vi "oa_Build Spectral Info (N Channels).vi"(0 "spectra in":dbl[][][](array[numeric]) format="%.2f", 1 "processing control in":T1(ring), 5 "channel info":T8[](array[typedef]) {"channel info"."pregain" format="%.2f"; "channel info"."weighting filter" items=["Linear", "A-weighting", "B-weighting", "C-weighting", "ITU-R 468-4", "Dolby", "CCITT", "C-message", "Wb", "Wc", "Wd", "We", "Wf", "Wh", "Wj", "Wk", "Wm", "AES17 20 kHz lowpass", "AES17 40 kHz lowpass", "AES17 20 kHz highpass", "AES17 40 kHz highpass"]; "channel info"."dB reference" format="%^.1e"; "channel info"."engineering units" items=["custom..."=0, "V"=1, "A"=21, "C"=30, "pC"=31, "s"=32, "-"=29, "Pa"=2, "N"=20, "g"=3, "m/s^2"=4, "m/s"=5, "m"=6, "mm/s"=12, "mm"=13, "micron/s"=14, "micron"=15, "in/s^2"=7, "in/s"=8, "in"=9, "mil/s"=10, "mil"=11, "rad/s^2"=16, "rad/s"=17, "rad"=18, "deg/s^2"=26, "deg/s"=27, "deg"=28, "RPM"=22, "cycle/s^2"=23, "Hz"=24, "cycle"=25, "strain"=19]; "channel info"."sensor sensitivity" format="%#_5f"}, 7 "spectrum settings":cluster{"window type":u16, "block size":i32}={"window type"=1, "block size"=400} {"block size" min=2; "window type" items=["None"=0, "Hanning"=1, "Hamming"=2, "Blackman-Harris"=3, "Exact Blackman"=4, "Blackman"=5, "Flat Top"=6, "4 Term B-Harris"=7, "7 Term B-Harris"=8, "Low Sidelobe"=9, "Gaussian"=62]}, 11 "error in":errorcluster, 12 "spectrum type":T4=enum."Power [Magnitude^2]") -> (2 "spectrum info":T2[](array[typedef]) {"x-axis units" items=["Time (s)"=0, "Frequency-CB (Hz)"=1, "Frequency-CPB (Hz)"=1248, "Frequency-Arbitrary (Hz)"=2357, "Quefrency (s)"=2, "Revolutions (rev)"=3, "Order"=4, "Speed (RPM)"=11, "Speed (rad/s)"=21, "Index"=65535]; "weighting filter" items=["Linear", "A-weighting", "B-weighting", "C-weighting", "ITU-R 468-4", "Dolby", "CCITT", "C-message", "Wb", "Wc", "Wd", "We", "Wf", "Wh", "Wj", "Wk", "Wm", "AES17 20 kHz lowpass", "AES17 40 kHz lowpass", "AES17 20 kHz highpass", "AES17 40 kHz highpass"]; "dB reference [EU]" format="%.2f"; "engineering units" items=["custom..."=0, "V"=1, "A"=21, "C"=30, "pC"=31, "s"=32, "-"=29, "Pa"=2, "N"=20, "g"=3, "m/s^2"=4, "m/s"=5, "m"=6, "mm/s"=12, "mm"=13, "micron/s"=14, "micron"=15, "in/s^2"=7, "in/s"=8, "in"=9, "mil/s"=10, "mil"=11, "rad/s^2"=16, "rad/s"=17, "rad"=18, "deg/s^2"=26, "deg/s"=27, "deg"=28, "RPM"=22, "cycle/s^2"=23, "Hz"=24, "cycle"=25, "strain"=19]; "spectral info"."window" items=["None "=0, "Hanning"=1, "Hamming"=2, "Blackman-Harris"=3, "Exact Blackman"=4, "Blackman"=5, "Flat Top"=6, "4 Term B-Harris "=7, "7 Term B-Harris"=8, "Low Sidelobe"=9, "Force - Exponential"=10, "Gaussian"=62]}, 3 "dup processing control":T1(ring), 4 "spectra out":dbl[][][](array[numeric]) format="%.2f", 15 "error out":errorcluster)   [LabVIEW 2017, in "SoundVib_Resampling.lvlib"]
uses:
  <vilib>/addons/Sound and Vibration/Order Analysis/Resample Order Tracking/SoundVib_Resampling.lvlib
  <vilib>/addons/_NISVFA/_Shared subVIs/Controls/svc_Resampled Channel Info.ctl
  <vilib>/addons/_NISVFA/_Shared subVIs/Controls/svc_Channel Info.ctl
  <vilib>/addons/_NISVFA/_Shared subVIs/Controls/svc_Engineering Units Text Ring.ctl
  <vilib>/addons/_NISVFA/_Shared subVIs/Controls/svc_Weighting Filter Text Ring.ctl
  <vilib>/addons/_NISVFA/_Shared subVIs/Controls/svc_Spectrum Type.ctl
  <vilib>/addons/_NISVFA/_Shared subVIs/Controls/svc_Spectrum Info.ctl
  <vilib>/addons/_NISVFA/_Shared subVIs/Controls/svc_X-Axis Units.ctl
  <vilib>/addons/_NISVFA/_Shared subVIs/Controls/svc_Complimentary Spectrum Units.ctl
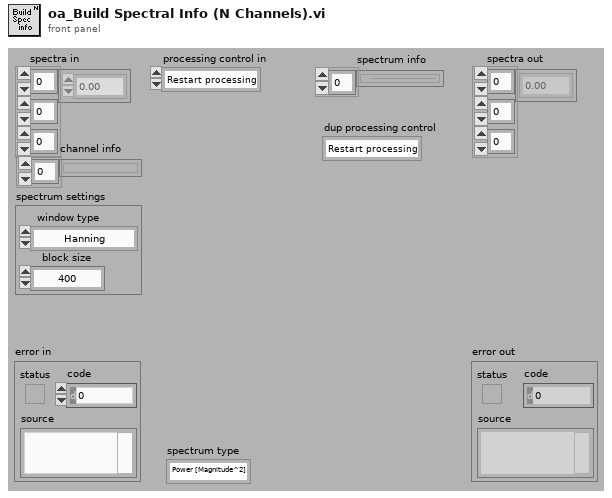
[diagram p1: front panel]
types:
  T1 = enum16{"Restart processing", "Continue processing", "Skip processing"}
  T2 = typedef "svc_Spectrum Info.ctl" = cluster{"channel name":string, "description":string, "x-axis units":T3, "spectral info":cluster{"spectrum type":T4, "linear/dB":enum16{"linear", "dB"}, "window":u16, "window size":i32, "FFT size":i32}, "engineering units":T5, "custom label":string, "dB reference [EU]":dbl, "peak units":enum16{"rms", "peak", "peak-peak"}, "weighting filter":T6, "spectral density?":bool, "unit label":string, "spectrum skewed?":bool, "complimentary spectrum units":T7}
  T3 = typedef "svc_X-Axis Units.ctl" = u16
  T4 = typedef "svc_Spectrum Type.ctl" = enum16{"FFT Spectrum [complex]", "Amplitude [Magnitude]", "Power [Magnitude^2]", "Cross Spectrum [complex]", "Frequency Response [Complex]"}
  T5 = typedef "svc_Engineering Units Text Ring.ctl" = u16
  T6 = typedef "svc_Weighting Filter Text Ring.ctl" = u16
  T7 = typedef "svc_Complimentary Spectrum Units.ctl" = enum16{"none", "radians", "degrees", "cycles", "imaginary"}
  T8 = typedef "svc_Resampled Channel Info.ctl" = cluster{"channel name":string, "description":string, " channel info":T9}
  T9 = typedef "svc_Channel Info.ctl" = cluster{"sensor sensitivity":dbl, "engineering units":T5, "dB reference":dbl, "custom label":string, "weighting filter":T6, "pregain":dbl}
  T10 = cluster{"spectrum type":T4, "linear/dB":enum16{"linear", "dB"}, "window":u16, "window size":i32, "FFT size":i32}
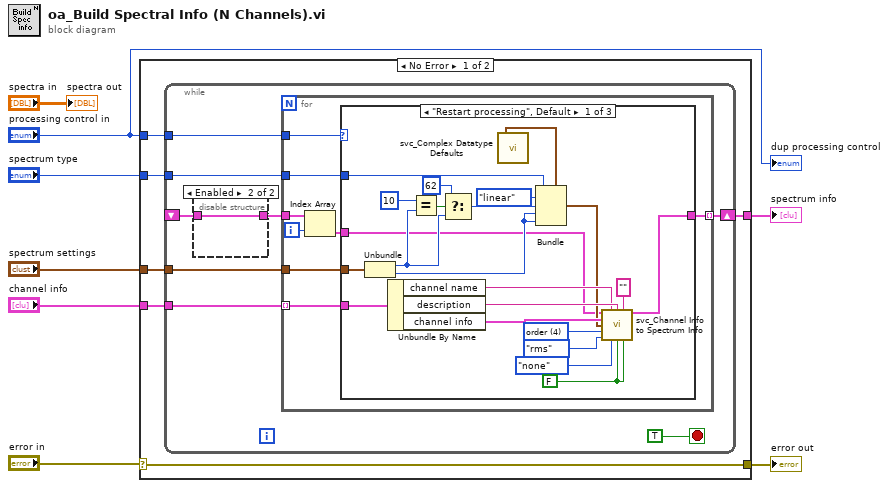
[diagram p0: block diagram]
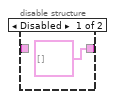
[diagram p2: hidden frame]
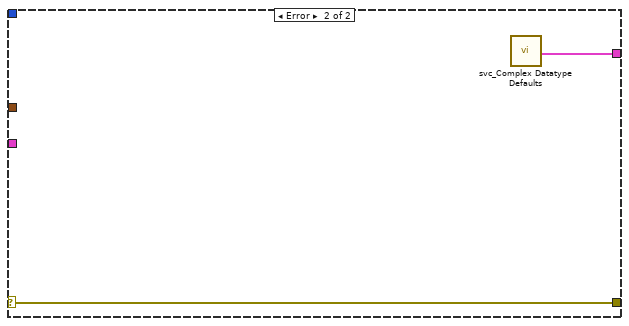
[diagram p5: hidden frame]
diagram:
  n1 = case shown="No Error" "error in" {
    selector: "error in" -> [w14 w58]
    tunnel: [w14 w58] -> w2
    tunnel: "processing control in" -> [w13 _]
    tunnel: [w9 w57] -> w4
    tunnel: "spectrum type" -> [w12 _]
    tunnel: "channel info" -> [w11 _]
    tunnel: "spectrum settings" -> [w10 _]
    frame No Error {
      n2 = while {
        tunnel: w13 -> [w22]
        shift-right: [w20] -> w9
        shift-left: _ -> [w15]
        tunnel: w12 -> [w19]
        tunnel: w11 -> [w18]
        tunnel: w10 -> [w17]
        stop <- TRUE stop-if-true
        n3 = disable-structure shown="Enabled" {
          disable-tunnel: [T2[] [] w24] -> w16
          disable-tunnel: w15 -> [_ w24]
          frame Disabled {
          }
          frame Enabled {
          }
        }
        n4 = for {
          tunnel: w22 -> [w32]
          tunnel: [w31] -> w20 mode=indexing
          tunnel: w16 -> [w26]
          tunnel: w19 -> [w30]
          tunnel: w18 -> [w29] mode=indexing
          tunnel: w17 -> [w28]
          i -> [w25]
          n5 = Index Array(array=w26, index=w25) -> (element=w27:T2)
          n6 = case shown="\"Restart processing\", Default" w32 {
            tunnel: [w52 w55 w56] -> w31
            tunnel: w27 -> [w34 w55 w56]
            tunnel: w30 -> [w45 _ _]
            tunnel: w29 -> [w53 _ _]
            tunnel: w28 -> [w54 _ _]
            frame "Restart processing", Default {
              w49 = FALSE ("spectral density?")
              w46 = u16 4 items=["time"=0, "frequency"=1, "quefrency"=2, "revolutions"=3, "order"=4, "rpm"=11] ("x-axis units")
              n7 = Unbundle(w54) -> ("window type"=w41:u16, "block size"=w48:i32)
              n8 = Unbundle By Name(w53) -> ("channel name"=w50:string, "description"=w51:string, "channel info"=w44:T9)
              n9 = Equal?(x=u16 10, y=w41) -> (x = y?=w42:bool)
              n10 = Select(t=u16 62 ("x"), s=w42, f=w41) -> (s? t:f=w39:u16)
              n11 = call <vilib>:"svc_Complex Datatype Defaults.vi"() -> ("spectral info"=w37:T10)  [unwired: 11 in, 8 out]
              n12 = Bundle(cluster=w37, "spectrum type"=w45, "linear/dB"=enum16{"linear", "dB"}."linear" ("spectral info.linear/dB"), "window"=w39, "window size"=w48, "FFT size"=w48) -> (w38:T10)
              n13 = call <vilib>:"svc_Channel Info to Spectrum Info.vi"("spectrum info in"=w34, "channel name"=w50, "description"=w51, "unit label"="", "channel info"=w44, "spectral info"=w38, "x-axis units"=w46, "peak units"=enum16{"rms", "peak", "peak-peak"}."rms", "complimentary spectrum units"=svc_Complimentary_Spectrum_Units."none", "spectral density?"=w49, "spectrum skewed?"=w49) -> ("spectrum info out"=w52:T2)  [unwired: 4 in]
            }
            frame "Continue processing" {
            }
            frame "Skip processing" {
            }
          }
        }
      }
    }
    frame Error {
      n14 = call <vilib>:"svc_Complex Datatype Defaults.vi"() -> ("empty array of spectrum info"=w57:T2[])  [unwired: 11 in, 8 out]
    }
  }
  "error out" <- w2
  "spectrum info" <- w4
  "spectra out" <- "spectra in"
  "dup processing control" <- "processing control in"
